vi "CT_CryoControlMultiInputs.vi"(0 "Vacuum Sensors":T3={"TP On"=FALSE, "IG1 On"=TRUE, "IG2On"=FALSE, "IG Vac Level"=7.206095277894153e-07, "CG1 Vac Level"=7.188197481794052e-05, "CG2 Vac Level"=7.698533430214743e-05, "IG Status"=TRUE} {"CG2 Vac Level" format="%#_2e"; "CG1 Vac Level" format="%#_2e"; "IG Vac Level" format="%#_2e"}, 1 "Turbo CG1 Thresh":dbl=9.9e-06 min=1e-10 max=0.0001, 3 "Charge Step":T4(ring), 5 "Cryo Thresh":dbl, 6 "Turbo Gate":bool=TRUE, 7 "Turbo IG Thresh":dbl=9.9e-06 min=1e-10 max=0.0001, 9 "Cryo 1 Gate":bool=TRUE, 11 "Cryo 2 Gate":bool=TRUE, 12 "Charge Cycle Done":bool caption="Charge\nDone", 13 "Running  \nShot \nSequence":bool, 14 "Puff High\nRef Shot":bool) -> (4 "Cryo 1 Ctrl":bool, 10 "Cryo 2 Ctrl":bool, 15 "Turbo Ctrl":bool)   [LabVIEW 2016]
uses:
  VacuumMeasurementControlState.ctl
panel:
  in  "Cryo Gate":T1(ring)
  in  "Ion Gauge":T2
  in  "Turbo Gate":T1(ring)
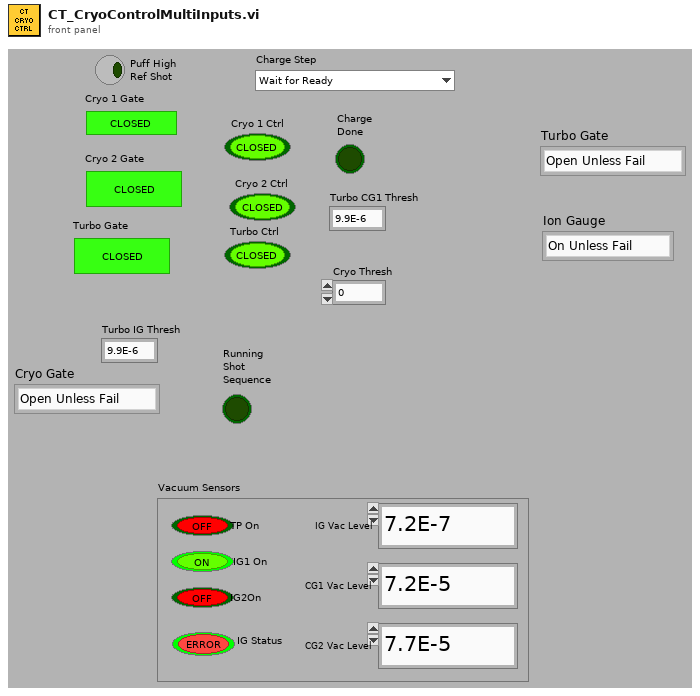
[diagram p1: front panel]
types:
  T1 = enum16{"Open Unless Fail", "Open Unless Shot", "Close"}
  T2 = typedef "VacuumMeasurementControlState.ctl" = enum16{"On Unless Fail", "On Unless Shot", "Force Off", "Manual"}
  T3 = cluster{"TP On":bool, "IG1 On":bool, "IG2On":bool, "IG Vac Level":dbl, "CG1 Vac Level":dbl, "CG2 Vac Level":dbl, "IG Status":bool}
  T4 = enum16{"Wait for Ready", "Prep for Charge", "Open Dump Relays", "Close Connect Relays", "Wait PS Delays", "Wait End of Charge", "Turn Off HV", "Open Connect Relays", "Charge Done"}
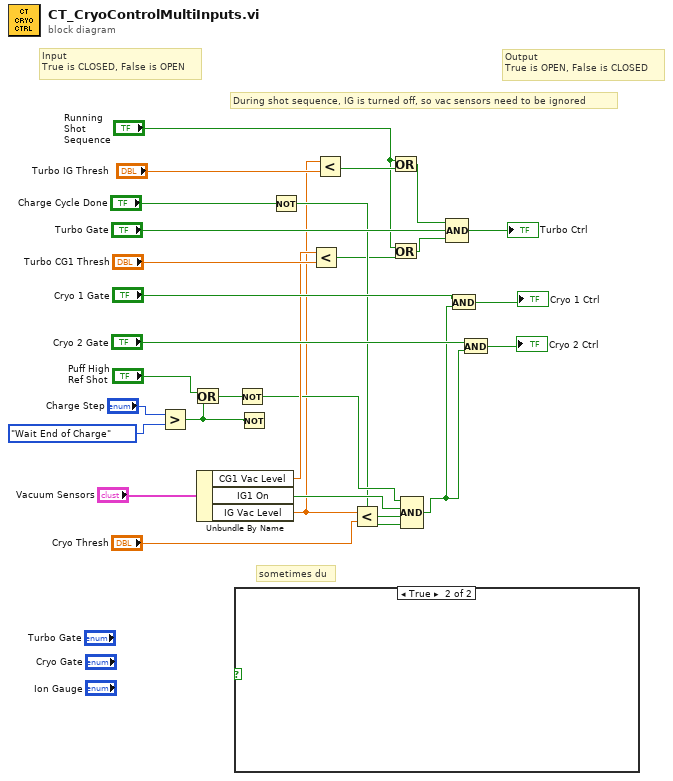
[diagram p0: block diagram]
diagram:
  # "sometimes du"
  # "During shot sequence, IG is turned off, so vac sensors need to be ignored"
  # "Input\nTrue is CLOSED, False is OPEN"
  # "Output\nTrue is OPEN, False is CLOSED"
  n1 = Greater?(x="Charge Step", y=T4."Wait End of Charge") -> (0:w19:bool)
  n2 = Or(x="Puff High\nRef Shot", y=w19) -> (x .or. y?=w21:bool)
  n3 = Unbundle By Name("Vacuum Sensors") -> ("CG1 Vac Level"=w15:dbl, "IG1 On"=w11:bool, "IG Vac Level"=w6:dbl)
  n4 = case shown="True" {
    selector: _ -> [_ _]
    frame False {
    }
    frame True {
    }
  }
  n5 = Not(x=w21) -> (.not. x?=w12:bool)
  n6 = Not(x=w19) -> ()  [unwired: 1 out]
  n7 = Not(x="Charge Cycle Done") -> (.not. x?=w9:bool)
  n8 = Less?(x=w15, y="Turbo CG1 Thresh") -> (x < y?=w3:bool)
  n9 = Less?(x=w6, y="Turbo IG Thresh") -> (x < y?=w5:bool)
  n10 = Less?(x=w6, y="Cryo Thresh") -> (x < y?=w10:bool)
  n11 = Or(x="Running  \nShot \nSequence", y=w5) -> (x .or. y?=w4:bool)
  n12 = Or(x="Running  \nShot \nSequence", y=w3) -> (x .or. y?=w2:bool)
  n13 = Compound Arithmetic op=AND(w12, w11, w10, w9) -> (w13:bool)
  n14 = Compound Arithmetic op=AND(w4, "Turbo Gate", w2) -> (→"Turbo Ctrl":bool)
  n15 = And(x="Cryo 1 Gate", y=w13) -> (x .and. y?=→"Cryo 1 Ctrl":bool)
  n16 = And(x="Cryo 2 Gate", y=w13) -> (x .and. y?=→"Cryo 2 Ctrl":bool)
